vi "Check Error.vi"(8 "Error in":errorcluster, 10 "Actor in":refnum<class "Actor.lvclass">) -> (2 "Actor out":refnum<class "Actor.lvclass">)   [LabVIEW 2020, in "jettl.lvlib" / "Actor.lvlib"]
uses:
  Actor.lvlib
  Actor/Actor.lvclass
  Go To Destroy Msg/Go To Destroy Msg.lvlib
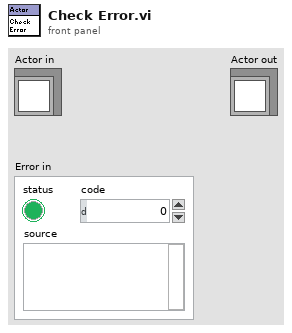
[diagram p1: front panel]
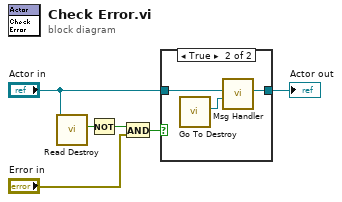
[diagram p0: block diagram]
diagram:
  n1 = call-dynamic "Read Destroy.vi"("Actor in"="Actor in") -> ("Destroy"=w4:bool)  [unwired: 10 in]
  n2 = Not(x=w4) -> (.not. x?=w3:bool)
  n3 = And(x=w3, y="Error in") -> (x .and. y?=w1:bool)
  n4 = case shown="True" w1 {
    tunnel: "Actor in" -> [w7 w10]
    tunnel: [w7 w8] -> w2
    frame False {
    }
    frame True {
      n5 = call "Go To Destroy.vi"() -> ("Msg"=w9:refnum<class "Msg.lvclass">)  [unwired: 11 in]
      n6 = call "Msg Handler.vi"("Msg"=w9, "Actor in"=w10) -> ("Actor out"=w8:refnum<class "Actor.lvclass">)  [unwired: 8 in, 1 out]
    }
  }
  "Actor out" <- w2
